vi "Total Archived Data.vi"(8 "Add Volts":bool, 9 "2 LBCB Archiving Mode":bool, 10 "Use Hold":bool, 11 "Number of LBCBs":T1) -> (0 "Combined":dbl[](array[numeric]), 1 "External Sensors":dbl[](array[numeric]), 2 "LBCB 2":dbl[](array[numeric]), 3 "LBCB 1":dbl[](array[numeric]))   [LabVIEW 2009]
uses:
  Data Access Objects/Metadata/DAO Actions.ctl
  Cartesian Measurment Actions.ctl
  Data Access Objects/Metadata/LBCB Number.ctl
  Data Access Objects/Application/Number Of LBCBs.ctl
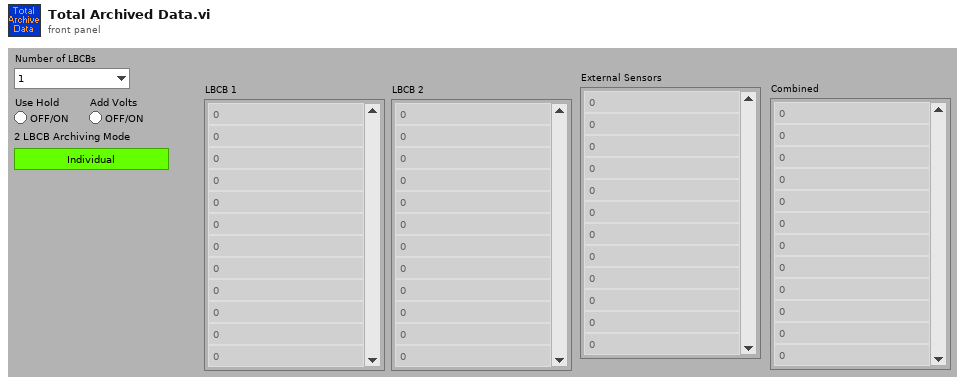
[diagram p1: front panel]
types:
  T1 = typedef "Number Of LBCBs.ctl" = enum16{"1", "2"}
  T2 = typedef "Cartesian Measurment Actions.ctl" = enum16{"Set Data", "Get", "Init", "Set Offsets"}
  T3 = typedef "LBCB Number.ctl" = enum16{"LBCB1", "LBCB2"}
  T4 = typedef "DAO Actions.ctl" = enum16{"Init", "Get", "Set"}
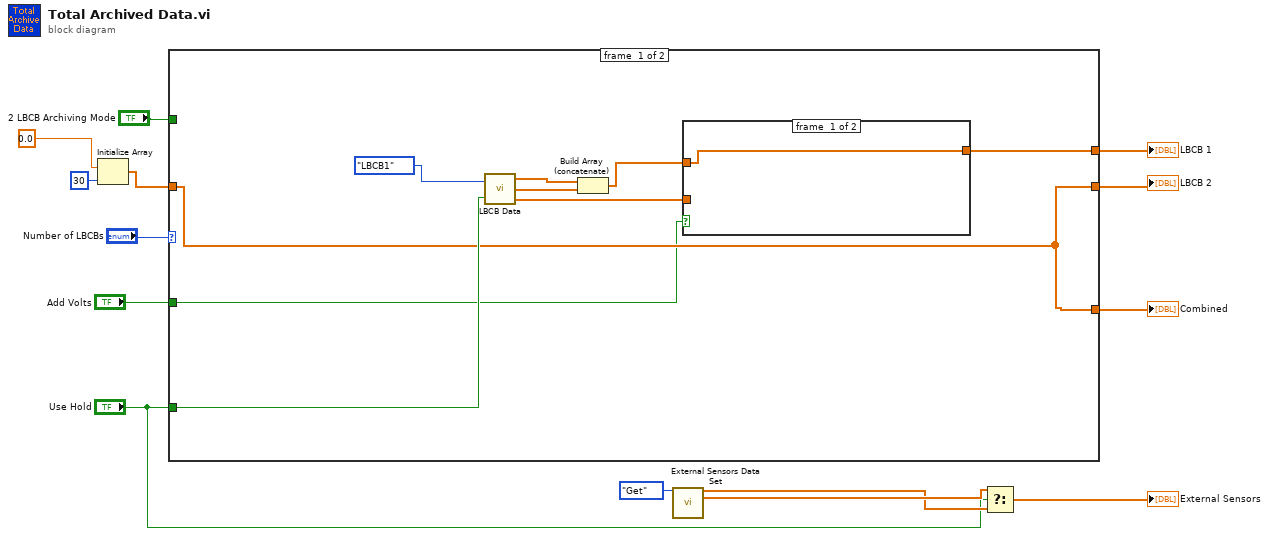
[diagram p0: block diagram]
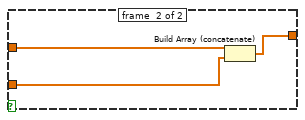
[diagram p2: hidden frame]
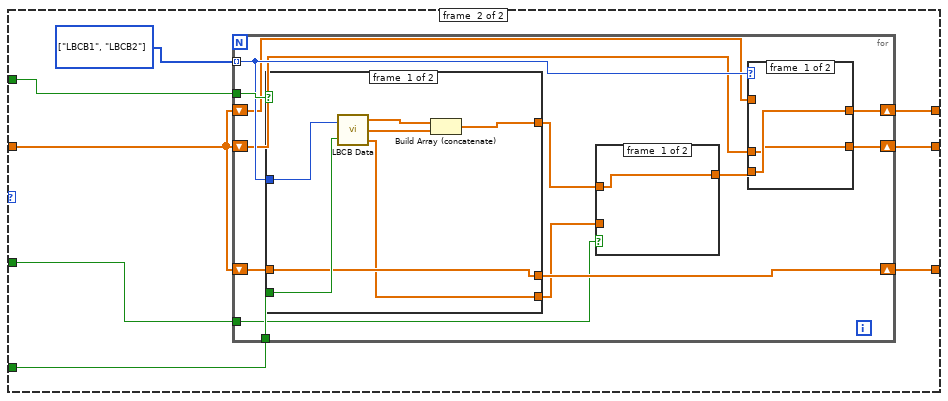
[diagram p3: hidden frame]
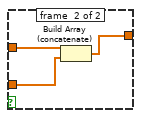
[diagram p4: hidden frame]
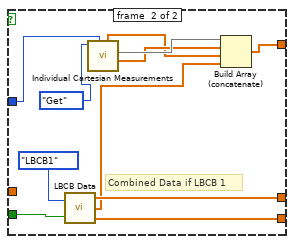
[diagram p6: hidden frame]
diagram:
  n1 = Initialize Array(0.0, 30 ("dimension size")) -> (w2:dbl[])
  n2 = case shown="\"2\"" "Number of LBCBs" {
    tunnel: "2 LBCB Archiving Mode" -> [_ w35]
    tunnel: "Use Hold" -> [w20 w34]
    tunnel: [w15 w32] -> w7
    tunnel: [w19 w31] -> w6
    tunnel: [w19 w30] -> w5
    tunnel: w2 -> [w19 w29]
    tunnel: "Add Volts" -> [w17 w28]
    frame #0 {
      n3 = call "LBCB Data.vi"("LBCB Number"=LBCB_Number."LBCB1", "Use Hold"=w20) -> ("Cart Data"=w23:dbl[], "Act Data"=w22:dbl[], "Act Volts"=w16:dbl[])
      n4 = Build Array (concatenate)(w23, w22) -> (w18:dbl[])
      n5 = case shown="False" w17 {
        tunnel: w18 -> [w24 w27]
        tunnel: w16 -> [_ w26]
        tunnel: [w24 w25] -> w15
        frame #0 {
        }
        frame #1 {
          n6 = Build Array (concatenate)(w27, w26) -> (w25:dbl[])
        }
      }
    }
    frame #1 {
      w33 = T3[] [enum."LBCB1", enum."LBCB2"] items=["LBCB1", "LBCB2"]
      n7 = for {
        tunnel: w35 -> [w48]
        tunnel: w34 -> [w47]
        tunnel: w33 -> [w44] mode=indexing
        shift-right: [w43] -> w32
        shift-left: w29 -> [w40]
        shift-right: [w41] -> w31
        shift-left: w29 -> [w42]
        shift-right: [w46] -> w30
        shift-left: w29 -> [w45]
        tunnel: w28 -> [w36]
        n8 = case shown="False" w48 {
          tunnel: w47 -> [w63 w74]
          tunnel: [w58 w68] -> w46
          tunnel: w44 -> [w62 w69]
          tunnel: [w60 w66] -> w39
          tunnel: w45 -> [w58 _]
          tunnel: [w57 w65] -> w37
          frame #0 {
            n9 = call "LBCB Data.vi"("LBCB Number"=w62, "Use Hold"=w63) -> ("Cart Data"=w61:dbl[], "Act Data"=w59:dbl[], "Act Volts"=w57:dbl[])
            n10 = Build Array (concatenate)(w61, w59) -> (w60:dbl[])
          }
          frame #1 {
            # "Combined Data if LBCB 1"
            n11 = call "LBCB Data.vi"("LBCB Number"=LBCB_Number."LBCB1", "Use Hold"=w74) -> ("Cart Data"=w68:dbl[], "Act Data"=w67:dbl[], "Act Volts"=w65:dbl[])
            n12 = call "Individual Cartesian Measurements.vi"("LBCB Number"=w69, "DAO Actions"=DAO_Actions."Get") -> ("Displacements Out"=w71:dbl[], 2:w72, "Forces Out"=w70:dbl[])  [unwired: 6 in, 1 out]
            n13 = Build Array (concatenate)(w72, w71, w70, w67) -> (w66:dbl[])
          }
        }
        n14 = case shown="True" w36 {
          tunnel: w39 -> [w49 w52]
          tunnel: w37 -> [_ w51]
          tunnel: [w49 w50] -> w38
          frame #0 {
          }
          frame #1 {
            n15 = Build Array (concatenate)(w52, w51) -> (w50:dbl[])
          }
        }
        n16 = case shown="\"LBCB2\"" w44 {
          tunnel: w38 -> [w54 w55]
          tunnel: [w54 w56] -> w43
          tunnel: w42 -> [w53 _]
          tunnel: [w53 w55] -> w41
          tunnel: w40 -> [_ w56]
          frame #0 {
          }
          frame #1 {
          }
        }
      }
    }
  }
  "LBCB 1" <- w7
  "LBCB 2" <- w6
  "Combined" <- w5
  n17 = call "External Sensors Data Set.vi"("Measurement Actions"=Cartesian_Measurment_Actions."Get") -> ("Data Out"=w11:dbl[], "Hold Data Out"=w12:dbl[])  [unwired: 10 in, 3 out]
  n18 = Select(t=w12, s="Use Hold", f=w11) -> (s? t:f=→"External Sensors":dbl[])
